vi "MGI Spline Interpolation with Derivative.vi"(3 "x value":dbl format="%.2f", 4 "Interpolant[]":dbl[](array[numeric]) format="%.2f", 5 "x[]":dbl[](array[numeric]) format="%.2f", 6 "y[]":dbl[](array[numeric]) format="%.2f") -> (0 "error":i32, 1 "first derivative":dbl format="%.2f", 2 "interpolation value":dbl format="%.2f")   [LabVIEW 2020]
doc: "Calculate spline and first derivative using pre-calculated interpolant.\n\n\nAuthored by David A. Moore\nsupport@mooregoodideas.com\nwww.mooregoodideas.com\n\nCopyright (c) 2010, Moore Good Ideas, Inc.\n\nAll rights reserved.\n\nRedistribution and use in source and binary forms, with or without modification, are permitted provided that the following conditions are met:\n\n * Redistributions of source code must retain the above copyright notice, this list of conditions and the following disclaimer.\n * Redistributions in binary form must reproduce the above copyright notice, this list of conditions and the following disclaimer in the documentation and/or other materials provided with the distribution.\n * Neither the name of Moore Good Ideas, Inc. nor the names of its contributors may be used to endorse or promote products derived from this software without specific prior written permission.\n\nTHIS SOFTWARE IS PROVIDED BY THE COPYRIGHT HOLDERS AND CONTRIBUTORS \"AS IS\" AND ANY EXPRESS OR IMPLIED WARRANTIES, INCLUDING, BUT NOT LIMITED TO, THE IMPLIED WARRANTIES OF MERCHANTABILITY AND FITNESS FOR A PARTICULAR PURPOSE ARE DISCLAIMED. IN NO EVENT SHALL THE COPYRIGHT OWNER OR CONTRIBUTORS BE LIABLE FOR ANY DIRECT, INDIRECT, INCIDENTAL, SPECIAL, EXEMPLARY, OR CONSEQUENTIAL DAMAGES (INCLUDING, BUT NOT LIMITED TO, PROCUREMENT OF SUBSTITUTE GOODS OR SERVICES; LOSS OF USE, DATA, OR PROFITS; OR BUSINESS INTERRUPTION) HOWEVER CAUSED AND ON ANY THEORY OF LIABILITY, WHETHER IN CONTRACT, STRICT LIABILITY, OR TORT (INCLUDING NEGLIGENCE OR OTHERWISE) ARISING IN ANY WAY OUT OF THE USE OF THIS SOFTWARE, EVEN IF ADVISED OF THE POSSIBILITY OF SUCH DAMAGE."
uses:
  <vilib>/Analysis/NI_AALPro.lvlib
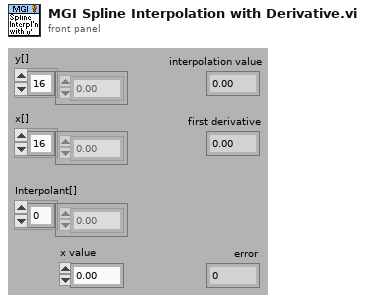
[diagram p1: front panel]
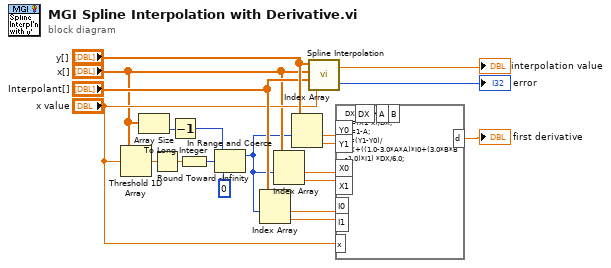
[diagram p0: block diagram]
diagram:
  n1 = Threshold 1D Array(2:"x value", 3:"x[]") -> (0:w18:dbl)  [unwired: 1 in]
  n2 = Array Size(array="x[]") -> (size(s)=w5:i32)
  n3 = Round Toward -Infinity(1:w18) -> (0:w7:dbl)
  n4 = Decrement(x=w5) -> (x-1=w2:i32)
  n5 = To Long Integer(number=w7) -> (32bit integer=w3:i32)
  n6 = In Range and Coerce(upper limit=w2, x=w3, lower limit=0) -> (coerced(x)=w4:i32)  [unwired: 1 out]
  n7 = Index Array(array="Interpolant[]", index #1=w4) -> (element #1=w11:dbl, element #2=w10:dbl)  [unwired: 1 in]
  n8 = Index Array(array="x[]", index #1=w4) -> (element #1=w13:dbl, element #2=w12:dbl)  [unwired: 1 in]
  n9 = Index Array(array="y[]", index #1=w4) -> (element #1=w15:dbl, element #2=w14:dbl)  [unwired: 1 in]
  n10 = call <vilib>:"Spline Interpolation.vi"("x value"="x value", "Interpolant"="Interpolant[]", "X"="x[]", "Y"="y[]") -> ("error"=→"error":i32, "interpolation value"=→"interpolation value":dbl)
  n11 = formula code="DX=X1-X0;\nA=(X1-x)/DX;\nB=1-A;\nd=(Y1-Y0)/DX+((1.0-3.0*A*A)*I0+(3.0*B*B-1.0)*I1) *DX/6.0;"("Y0"=w15, "Y1"=w14, "X0"=w13, "X1"=w12, "I0"=w11, "I1"=w10, "x"="x value") -> ("d"=→"first derivative":dbl)  [unwired: 3 out]
